vi "PH_Beckhoff_PP_PU.panel.vi"(0 "object ref":refnum<vi>, 5 "error in (no error)":errorcluster) -> (19 "error out":errorcluster)   [LabVIEW 2014, in "PH_Beckhoff_PP_PU.lvlib"]
doc: "This a GUI.\n\nLicense Agreement for this software:\n\nCopyright (C)\nGesellschaft für Schwerionenforschung, GSI\nPlanckstr. 1\n64291 Darmstadt\nGermany\n\nContact: D.Beck@gsi.de \n\nThis program is free software; you can redistribute it and/or modify it under the terms of the GNU General Public License as published by the Free Software Foundation; either version 2 of the license, or (at your option) any later version.\n\nThis program is distributed in the hope that it will be useful, but WITHOUT ANYW ARRANTY; without even the implied warranty of MERCHANTABILITY or FITNESS FOR A PARTICULAR PURPOSE. See the GNU General License for more details (http://www.gnu.org).\n\nGesellschaft für Schwerionenforschung, GSI\nPlanckstr. 1, 64291 Darmstadt, Germany\nFor all questions and ideas contact: M.Richter@gsi.de, H.Brand@gsi.de or D.Beck@gsi.de.\nLast update: 18-DEC-2002"
uses:
  PH_Beckhoff_PP_PU.lvlib
  PH_Beckhoff/PH_Beckhoff.Connectivity.ctl
  PH_Beckhoff/PH_Beckhoff.ADS Error.ctl
  PH_Beckhoff/PH_Beckhoff.Values.ctl
  PH_Beckhoff/PH_Beckhoff.Sonderklemmen Inputs.ctl
  PH_Beckhoff/PH_Beckhoff.Analog Inputs.ctl
  PH_Beckhoff/PH_Beckhoff.Scaling Type.ctl
  PH_Beckhoff/PH_Beckhoff.Analog Outputs.ctl
  PH_Beckhoff/PH_Beckhoff.Digital Inputs.ctl
  PH_Beckhoff/PH_Beckhoff.Digital Outputs.ctl
  PH_Beckhoff_PP_PU.PU Rack Type.ctl
  PH_StatusHandler/PH_StatusHandler.GUI element.ctl
  PH_PP_Common/PH_PP_Common.PSU Type.ctl
  PH_Beckhoff/PH_Beckhoff.GUI Refs.ctl
  CSCore/CSObj/CSObj.lvlib
  PH_Common/PH_Common.lvlib
  PH_Beckhoff/PH_Beckhoff.lvlib
  CSCore/CSSystem/CSSystemLib/CSSystemLib.lvlib
  PH_Class/PH_Class.lvlib
  PH_PP_Common/PH_PP_Common.lvlib
  PH_StatusHandler/PH_StatusHandler.lvlib
panel:
  in  "Tab Control":T1(tab)=enum."PUs ..."
  out "Current Values":T2
  in  "Show Info":bool
  out "configured?":bool
  out "Prdc Int [ms]":i32
  out "Connection":T9
  out "IP":string
  out "ADS Error":T10
  out "PU Rack Type":T11
  out "successfully \nreconfigured":i32=-1
  out "Trigger 2 Indicator":T13={"_Status"=0, "_triggered"=16860, "_fired"=16860, "last shot:"="no info available"} caption="_Trigger 2 ..."
  in  "_Ross close 2":bool caption="Ross 2 close"
  out "Ross 2 Indicator":T14={"_Status"=0, "_closed"=16860, "_open"=16860} caption="_Ross 2 ..."
  in  "_Device_on Ignitron 2":bool caption="Igni 2 Device-on"
  out "Ignitron 2 Indicator":T15={"_Status"=0, "_heating-on"=16860, "_water-on"=16860} caption="_Igni 2 ..."
  in  "_HV_on PSU 2":bool caption="PSU 2_HV_on"
  in  "_interlock_on PSU 2":bool caption="PSU 2_interlock_on"
  in  "_inhibit_on PSU 2":bool caption="PSU 2_inhibit_on"
  in  "_set_voltage PSU 2":dbl caption="PSU 2_voltage_set" format="%#_5g"
  out "Unit Voltage 2":string caption="V"
  out "PSU 2 Indicator":T16={"_Status"=0, "_inhibit_indicator"=16860, "_end_of_charge"=16860, "_HV_on"=16860, "_overtemperature"=16860, "_interlock_indicator"=16860, "_load_fault"=16860, "_sum_fault"=16860, "_HV_off"=16860, "_DC_ok"=16860, "_voltage_monitor"=0.0, "_current_monitor"=0.0} caption="_PSU 2 ..." {"_current_monitor" format="%#_5g"; "_voltage_monitor" format="%#_5g"}
  out "_voltage 2":dbl caption="_HV Meas 2" format="%#_7f"
  out "Unit HV Meas 2":string caption="V"
  out "Trigger 1 Indicator":T13={"_Status"=0, "_triggered"=16860, "_fired"=16860, "last shot:"="no info available"} caption="_Trigger 1 ..."
  in  "_Ross close 1":bool caption="Ross 1 close"
  out "Ross 1 Indicator":T14={"_Status"=0, "_closed"=16860, "_open"=16860} caption="_Ross 1 ..."
  in  "_Device_on Ignitron 1":bool caption="Igni 1 Device-on"
  out "Ignitron 1 Indicator":T15={"_Status"=0, "_heating-on"=16860, "_water-on"=16860} caption="_Igni 1 ..."
  in  "_HV_on PSU 1":bool caption="PSU 1_HV_on"
  in  "_interlock_on PSU 1":bool caption="PSU 1_interlock_on"
  in  "_inhibit_on PSU 1":bool caption="PSU 1_inhibit_on"
  out "PSU 1 Indicator":T16={"_Status"=0, "_inhibit_indicator"=16860, "_end_of_charge"=16860, "_HV_on"=16860, "_overtemperature"=16860, "_interlock_indicator"=16860, "_load_fault"=16860, "_sum_fault"=16860, "_HV_off"=16860, "_DC_ok"=16860, "_voltage_monitor"=0.0, "_current_monitor"=0.0} caption="_PSU 1 ..." {"_current_monitor" format="%#_5g"; "_voltage_monitor" format="%#_5g"}
  out "_voltage 1":dbl caption="_HV Meas 1" format="%#_7f"
  out "Unit HV Meas 1":string caption="V"
  in  "_set_voltage PSU 1":dbl caption="PSU 1_voltage_set" format="%#_5g"
  out "Unit Voltage 1":string caption="V"
  in  "_reset PSU 1":bool caption="PSU 1_reset"
  in  "_reset PSU 2":bool caption="PSU 2_reset"
  out "Type PSU 1":T17
  out "Type PSU 2":T17
  out "Limits 1 [V]":cluster{"Lower":dbl, "Upper":dbl}
  out "Limits 2 [V]":cluster{"Lower":dbl, "Upper":dbl}
  in  "Delete":bool
  in  "Exit":bool
  # "PCS"
  # "3.40"
  # "Pay attention! Commands are remote controlled! Handle with care!"
  # "A"
  # "V"
  # "A"
  # "V"
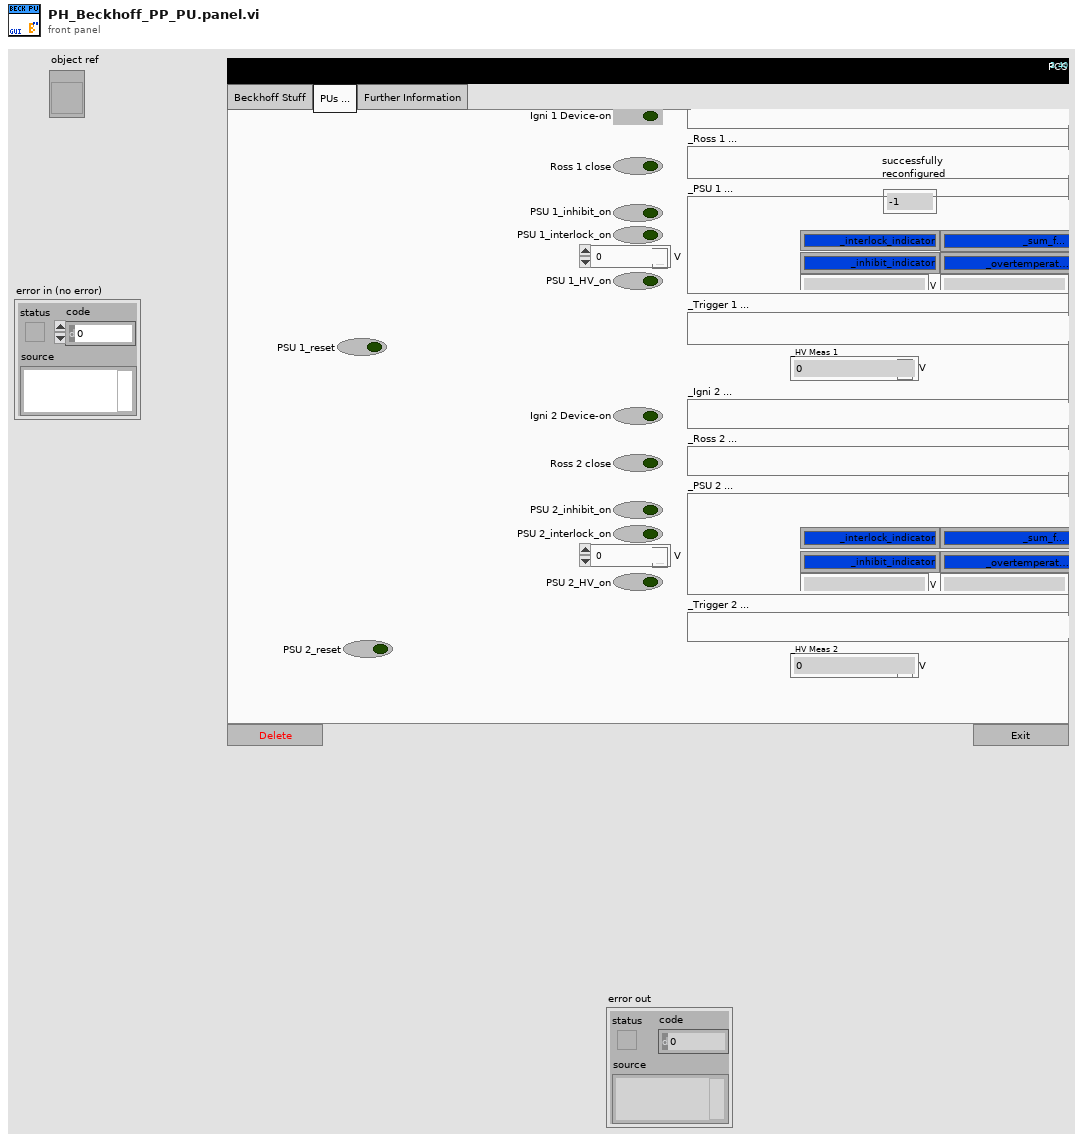
[diagram p1: front panel]
types:
  T1 = enum32{"Beckhoff Stuff", "PUs ...", "Further Information"}
  T2 = typedef "PH_Beckhoff.lvlib/PH_Beckhoff.Values.ctl" = cluster{"Sonderklemmen Inputs":T3, "Analog Inputs":T4, "Analog Outputs":T6, "Digital Inputs":T7, "Digital Outputs":T8}
  T3 = typedef "PH_Beckhoff.lvlib/PH_Beckhoff.Sonderklemmen Inputs.ctl" = cluster{"Total Length":u32, "Name":string, "Value":u64, "Quality":bool, "Service ID":i32, "Offset":u32, "Length":u32}[]
  T4 = typedef "PH_Beckhoff.lvlib/PH_Beckhoff.Analog Inputs.ctl" = cluster{"Name":string, "Value":u32, "Quality":bool, "Service ID":i32, "Sca Type":T5}[]
  T5 = typedef "PH_Beckhoff.lvlib/PH_Beckhoff.Scaling Type.ctl" = enum16{"none", "0 ... 15 Bit -> 0 ... 5", "0 ... 15 Bit -> 0 ... 10", "0 ... 15 Bit -> 0 ... 25", "0 ... 15 Bit -> 4 ... 20", "0 ... 15 Bit -> 0 ... 1", "0 ... 15 Bit -> 0 ... 20000", "0 ... 15 Bit -> 0 ... 24000"}
  T6 = typedef "PH_Beckhoff.lvlib/PH_Beckhoff.Analog Outputs.ctl" = cluster{"Name":string, "Value":u32, "Quality":bool, "Wanted Value":u32, "Service ID":i32, "Sca Type":T5}[]
  T7 = typedef "PH_Beckhoff.lvlib/PH_Beckhoff.Digital Inputs.ctl" = cluster{"Name":string, "Value":bool, "Quality":bool, "Service ID":i32, "inverted?":bool}[]
  T8 = typedef "PH_Beckhoff.lvlib/PH_Beckhoff.Digital Outputs.ctl" = cluster{"Name":string, "Value":bool, "Quality":bool, "Wanted Value":bool, "Service ID":i32, "inverted?":bool}[]
  T9 = typedef "PH_Beckhoff.lvlib/PH_Beckhoff.Connectivity.ctl" = cluster{"DLL?":bool, "Port?":bool, "Client?":bool, "Ping?":bool, "unsuccessful Pings":u32}
  T10 = typedef "PH_Beckhoff.lvlib/PH_Beckhoff.ADS Error.ctl" = cluster{"Latest Error":string, "Error List":string[]}
  T11 = typedef "PH_Beckhoff_PP_PU.lvlib/PH_Beckhoff_PP_PU.PU Rack Type.ctl" = enum16{"no Info", "PA 19mm", "PA 45mm", "MA PU 1 and 2", "MA PU 3 and 4", "MA PU 5 and 6", "MA FR and PILC"}
  T12 = typedef "PH_StatusHandler.lvlib/PH_StatusHandler.GUI element.ctl" = u16
  T13 = cluster{"_Status":T12, "_triggered":u32, "_fired":u32, "last shot:":string}
  T14 = cluster{"_Status":T12, "_closed":u32, "_open":u32}
  T15 = cluster{"_Status":T12, "_heating-on":u32, "_water-on":u32}
  T16 = cluster{"_Status":T12, "_inhibit_indicator":u32, "_end_of_charge":u32, "_HV_on":u32, "_overtemperature":u32, "_interlock_indicator":u32, "_load_fault":u32, "_sum_fault":u32, "_HV_off":u32, "_DC_ok":u32, "_voltage_monitor":dbl, "_current_monitor":dbl}
  T17 = typedef "PH_PP_Common.lvlib/PH_PP_Common.PSU Type.ctl" = enum16{"none", "Maxwell Standard", "DEL", "Maxwell ALE", "Continuum 601k"}
  T18 = typedef "PH_Beckhoff.lvlib/PH_Beckhoff.GUI Refs.ctl" = cluster{"ADS Error":refnum<vi>, "Values":refnum<vi>, "configured?":refnum<vi>, "Connection":refnum<vi>, "IP":refnum<vi>, "Prdc Int [ms]":refnum<vi>}
  T19 = typedef "PH_Beckhoff.lvlib/PH_Beckhoff.i attribute.ctl" = cluster{"GUI Refs":T18, "operation?":bool, "Default Prdc Interval":i32, "Connection":T9, "AMS Net ID":T20, "Klemmencluster: # of":T21, "Values":T2, "IP":string, "Description":string, "configured?":bool, "Change Manager":cluster{"Detemination wanted?":bool, "Values changed at":cluster{"Sonderklemmen Inputs":i32[], "Analog Inputs":i32[], "Analog Outputs":i32[], "Digital Inputs":i32[], "Digital Outputs":i32[]}}, "Difference to handle an analog input as change":u32}
  T20 = typedef "Beckhoff - Driver np.lvlib/Beckhoff Access.ctl" = cluster{"DLL path":path, "AMS Net ID":cluster{"1st # of IP":u8, "2nd # of IP":u8, "3rd # of IP":u8, "4th # of IP":u8, "In Port":u8, "Out Port":u8}}
  T21 = typedef "Beckhoff - Driver np.lvlib/Klemmendeclarer.ctl" = cluster{"Offset due to Sonderklemms":u32, "analog Inputs":u32, "analog Outputs":u32, "digital Input Bits":u32, "digital Output Bits":u32}
  T22 = typedef "PH_PP_Common.lvlib/PH_PP_Common.PUs.ctl" = enum16{"no Info", "PA-19mm-1", "PA-19mm-2", "PA-45mm-PILC", "PA-45mm-MAIN", "MA-PU-1", "MA-PU-2", "MA-PU-3", "MA-PU-4", "MA-PU-5", "MA-PU-6", "MA-FR", "MA-PILC", "PA-45mm-DP"}
  T23 = typedef "PH_Beckhoff_PP_PU.lvlib/PH_Beckhoff_PP_PU.i attribute.ctl" = cluster{"HV Meas":cluster{"Input GUI Ref":refnum<vi>, "Voltage Service ID":i32, "Voltage [V]":dbl, "Quality":bool, "# in Data":i32}[], "Trigger":cluster{"Status":cluster{"GUI Ref":refnum<vi>, "Status Service ID":i32, "Status":T24}, "last shot:":cluster{"GUI Ref":refnum<vi>, "Service ID":i32, "Time":string}, "DIs":cluster{"triggered":cluster{"GUI Ref":refnum<vi>, "# in Data":i32}, "fired":cluster{"GUI Ref":refnum<vi>, "# in Data":i32}}, "GUI Ref Indicator":refnum<vi>}[], "RR":cluster{"Status":cluster{"GUI Ref":refnum<vi>, "Status Service ID":i32, "Status":T24}, "DIs":cluster{"closed":cluster{"GUI Ref":refnum<vi>, "# in Data":i32}, "open":cluster{"GUI Ref":refnum<vi>, "# in Data":i32}}, "Close":cluster{"GUI Ref":refnum<vi>, "# in Data":i32}, "GUI Ref Indicator":refnum<vi>}[], "Igni":cluster{"Status":cluster{"GUI Ref":refnum<vi>, "Status Service ID":i32, "Status":T24}, "DIs":cluster{"heating on":cluster{"GUI Ref":refnum<vi>, "# in Data":i32}, "water on":cluster{"GUI Ref":refnum<vi>, "# in Data":i32}}, "Device on":cluster{"GUI Ref":refnum<vi>, "# in Data":i32}, "GUI Ref Indicator":refnum<vi>}[], "PSU":cluster{"Status":cluster{"GUI Ref":refnum<vi>, "Status Service ID":i32, "Status":T24}, "Limit Service ID":i32, "DIs":cluster{"inhibit":cluster{"GUI Ref":refnum<vi>, "# in Data":i32}, "end of charge":cluster{"GUI Ref":refnum<vi>, "# in Data":i32}, "HV on":cluster{"GUI Ref":refnum<vi>, "# in Data":i32}, "overtemp":cluster{"GUI Ref":refnum<vi>, "# in Data":i32}, "interlock":cluster{"GUI Ref":refnum<vi>, "# in Data":i32}, "load fault":cluster{"GUI Ref":refnum<vi>, "# in Data":i32}, "sum fault":cluster{"GUI Ref":refnum<vi>, "# in Data":i32}, "HV off":cluster{"GUI Ref":refnum<vi>, "# in Data":i32}, "DC ok":cluster{"GUI Ref":refnum<vi>, "# in Data":i32}}, "AIs":cluster{"voltage":cluster{"GUI Ref":refnum<vi>, "# in Data":i32}, "current":cluster{"GUI Ref":refnum<vi>, "# in Data":i32}}, "DAs":cluster{"inhibit":cluster{"GUI Ref":refnum<vi>, "# in Data":i32}, "interlock":cluster{"GUI Ref":refnum<vi>, "# in Data":i32}, "HV on":cluster{"GUI Ref":refnum<vi>, "# in Data":i32}, "Reset":cluster{"GUI Ref":refnum<vi>, "# in Data":i32}}, "AAs":cluster{"Voltage to set":cluster{"GUI Ref":refnum<vi>, "# in Data":i32}}, "GUI Ref Indicator":refnum<vi>}[], "reconfigured":cluster{"?":bool, "GUI Ref":refnum<vi>}, "PU Rack Type":T11, "HV Meas Info":T25, "PSU Info":T26}
  T24 = typedef "PH_StatusHandler.lvlib/PH_StatusHandler.Status.ctl" = i16
  T25 = typedef "PH_Beckhoff_PP_PU.lvlib/PH_Beckhoff_PP_PU.HV Meas Info.ctl" = cluster{"Period Time [s]":dbl, "Subtractor 1 [Hz]":dbl, "Devider 1 [Hz/kV]":dbl, "Subtractor 2 [Hz]":dbl, "Devider 2 [Hz/kV]":dbl}
  T26 = typedef "PH_Beckhoff_PP_PU.lvlib/PH_Beckhoff_PP_PU.PSU Info.ctl" = cluster{"Limits 1 [V]":cluster{"Lower":dbl, "Upper":dbl}, "Limits 2 [V]":cluster{"Lower":dbl, "Upper":dbl}}
  T27 = cluster{"Status":cluster{"GUI Ref":refnum<vi>, "Status Service ID":i32, "Status":T24}, "DIs":cluster{"heating on":cluster{"GUI Ref":refnum<vi>, "# in Data":i32}, "water on":cluster{"GUI Ref":refnum<vi>, "# in Data":i32}}, "Device on":cluster{"GUI Ref":refnum<vi>, "# in Data":i32}, "GUI Ref Indicator":refnum<vi>}[]
  T28 = cluster{"Status":cluster{"GUI Ref":refnum<vi>, "Status Service ID":i32, "Status":T24}, "DIs":cluster{"closed":cluster{"GUI Ref":refnum<vi>, "# in Data":i32}, "open":cluster{"GUI Ref":refnum<vi>, "# in Data":i32}}, "Close":cluster{"GUI Ref":refnum<vi>, "# in Data":i32}, "GUI Ref Indicator":refnum<vi>}[]
  T29 = cluster{"Status":cluster{"GUI Ref":refnum<vi>, "Status Service ID":i32, "Status":T24}, "last shot:":cluster{"GUI Ref":refnum<vi>, "Service ID":i32, "Time":string}, "DIs":cluster{"triggered":cluster{"GUI Ref":refnum<vi>, "# in Data":i32}, "fired":cluster{"GUI Ref":refnum<vi>, "# in Data":i32}}, "GUI Ref Indicator":refnum<vi>}[]
  T30 = cluster{"Input GUI Ref":refnum<vi>, "Voltage Service ID":i32, "Voltage [V]":dbl, "Quality":bool, "# in Data":i32}[]
  T31 = cluster{"Status":cluster{"GUI Ref":refnum<vi>, "Status Service ID":i32, "Status":T24}, "Limit Service ID":i32, "DIs":cluster{"inhibit":cluster{"GUI Ref":refnum<vi>, "# in Data":i32}, "end of charge":cluster{"GUI Ref":refnum<vi>, "# in Data":i32}, "HV on":cluster{"GUI Ref":refnum<vi>, "# in Data":i32}, "overtemp":cluster{"GUI Ref":refnum<vi>, "# in Data":i32}, "interlock":cluster{"GUI Ref":refnum<vi>, "# in Data":i32}, "load fault":cluster{"GUI Ref":refnum<vi>, "# in Data":i32}, "sum fault":cluster{"GUI Ref":refnum<vi>, "# in Data":i32}, "HV off":cluster{"GUI Ref":refnum<vi>, "# in Data":i32}, "DC ok":cluster{"GUI Ref":refnum<vi>, "# in Data":i32}}, "AIs":cluster{"voltage":cluster{"GUI Ref":refnum<vi>, "# in Data":i32}, "current":cluster{"GUI Ref":refnum<vi>, "# in Data":i32}}, "DAs":cluster{"inhibit":cluster{"GUI Ref":refnum<vi>, "# in Data":i32}, "interlock":cluster{"GUI Ref":refnum<vi>, "# in Data":i32}, "HV on":cluster{"GUI Ref":refnum<vi>, "# in Data":i32}, "Reset":cluster{"GUI Ref":refnum<vi>, "# in Data":i32}}, "AAs":cluster{"Voltage to set":cluster{"GUI Ref":refnum<vi>, "# in Data":i32}}, "GUI Ref Indicator":refnum<vi>}[]
  T32 = cluster{"Status":cluster{"GUI Ref":refnum<vi>, "Status Service ID":i32, "Status":T24}, "Limit Service ID":i32, "DIs":cluster{"inhibit":cluster{"GUI Ref":refnum<vi>, "# in Data":i32}, "end of charge":cluster{"GUI Ref":refnum<vi>, "# in Data":i32}, "HV on":cluster{"GUI Ref":refnum<vi>, "# in Data":i32}, "overtemp":cluster{"GUI Ref":refnum<vi>, "# in Data":i32}, "interlock":cluster{"GUI Ref":refnum<vi>, "# in Data":i32}, "load fault":cluster{"GUI Ref":refnum<vi>, "# in Data":i32}, "sum fault":cluster{"GUI Ref":refnum<vi>, "# in Data":i32}, "HV off":cluster{"GUI Ref":refnum<vi>, "# in Data":i32}, "DC ok":cluster{"GUI Ref":refnum<vi>, "# in Data":i32}}, "AIs":cluster{"voltage":cluster{"GUI Ref":refnum<vi>, "# in Data":i32}, "current":cluster{"GUI Ref":refnum<vi>, "# in Data":i32}}, "DAs":cluster{"inhibit":cluster{"GUI Ref":refnum<vi>, "# in Data":i32}, "interlock":cluster{"GUI Ref":refnum<vi>, "# in Data":i32}, "HV on":cluster{"GUI Ref":refnum<vi>, "# in Data":i32}, "Reset":cluster{"GUI Ref":refnum<vi>, "# in Data":i32}}, "AAs":cluster{"Voltage to set":cluster{"GUI Ref":refnum<vi>, "# in Data":i32}}, "GUI Ref Indicator":refnum<vi>}
  T33 = cluster{"Status":cluster{"GUI Ref":refnum<vi>, "Status Service ID":i32, "Status":T24}, "DIs":cluster{"heating on":cluster{"GUI Ref":refnum<vi>, "# in Data":i32}, "water on":cluster{"GUI Ref":refnum<vi>, "# in Data":i32}}, "Device on":cluster{"GUI Ref":refnum<vi>, "# in Data":i32}, "GUI Ref Indicator":refnum<vi>}
  T34 = cluster{"Status":cluster{"GUI Ref":refnum<vi>, "Status Service ID":i32, "Status":T24}, "DIs":cluster{"closed":cluster{"GUI Ref":refnum<vi>, "# in Data":i32}, "open":cluster{"GUI Ref":refnum<vi>, "# in Data":i32}}, "Close":cluster{"GUI Ref":refnum<vi>, "# in Data":i32}, "GUI Ref Indicator":refnum<vi>}
  T35 = cluster{"Status":cluster{"GUI Ref":refnum<vi>, "Status Service ID":i32, "Status":T24}, "last shot:":cluster{"GUI Ref":refnum<vi>, "Service ID":i32, "Time":string}, "DIs":cluster{"triggered":cluster{"GUI Ref":refnum<vi>, "# in Data":i32}, "fired":cluster{"GUI Ref":refnum<vi>, "# in Data":i32}}, "GUI Ref Indicator":refnum<vi>}
  T36 = cluster{"Input GUI Ref":refnum<vi>, "Voltage Service ID":i32, "Voltage [V]":dbl, "Quality":bool, "# in Data":i32}
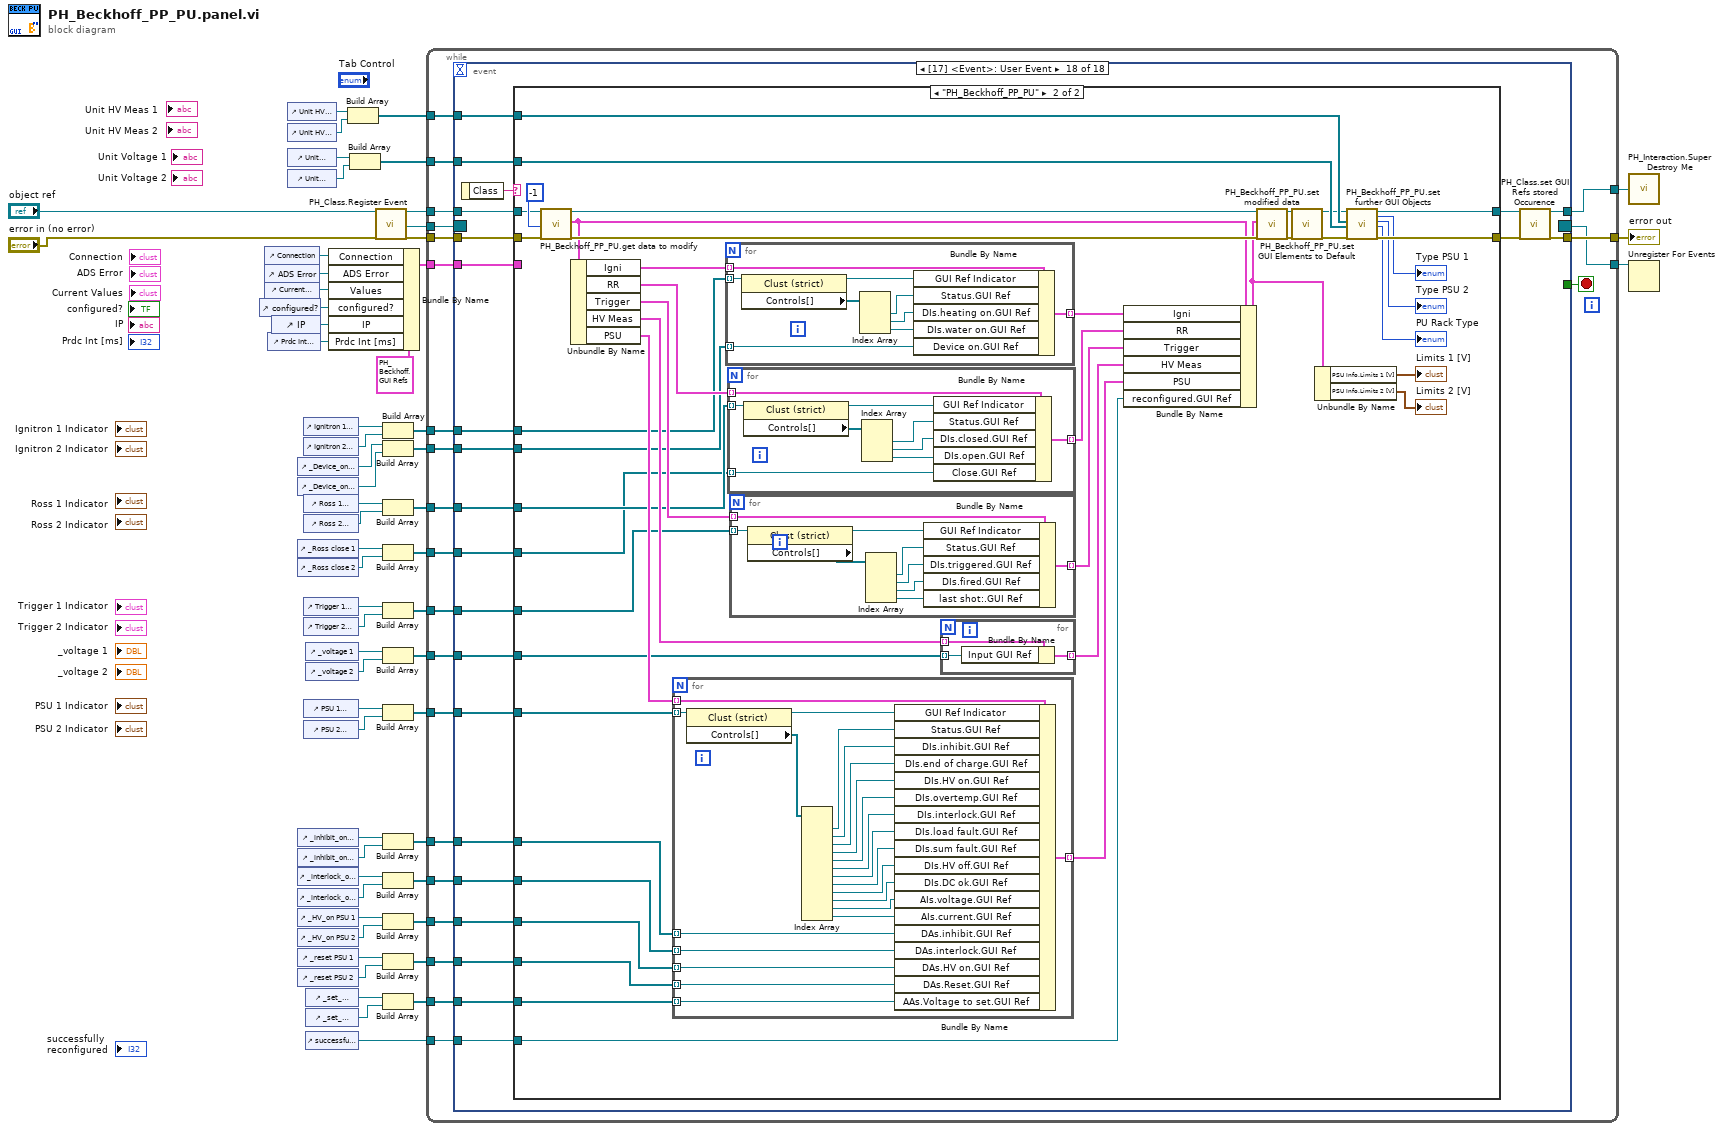
[diagram p0: block diagram]
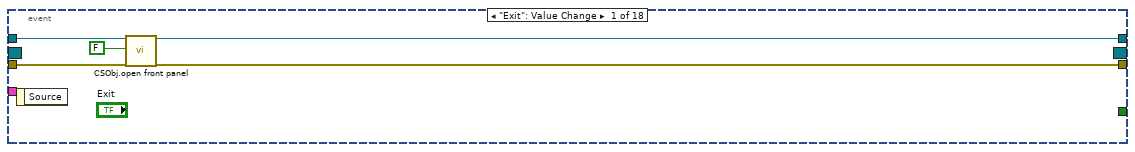
[diagram p2: hidden frame]
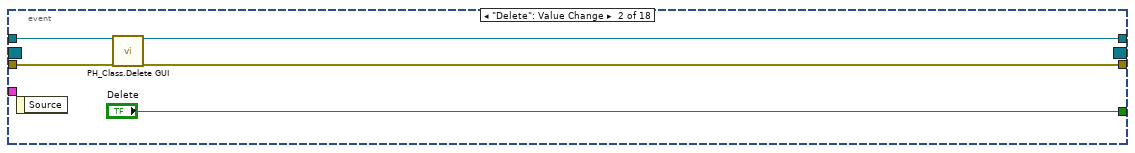
[diagram p3: hidden frame]
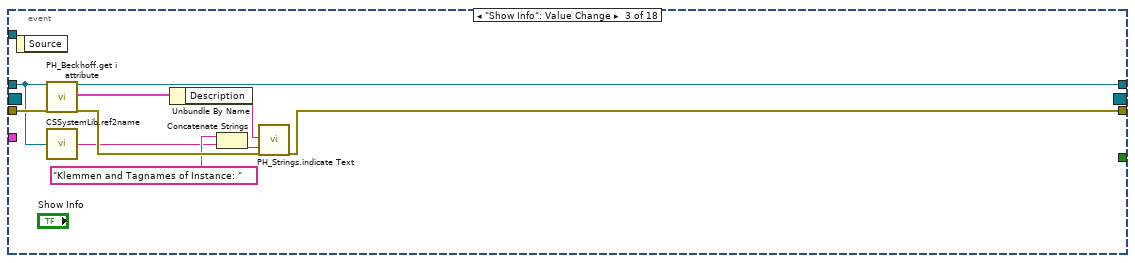
[diagram p4: hidden frame]
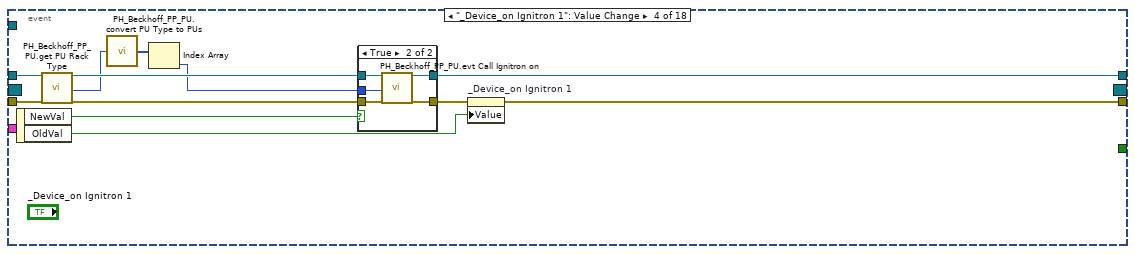
[diagram p5: hidden frame]
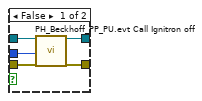
[diagram p6: hidden frame]
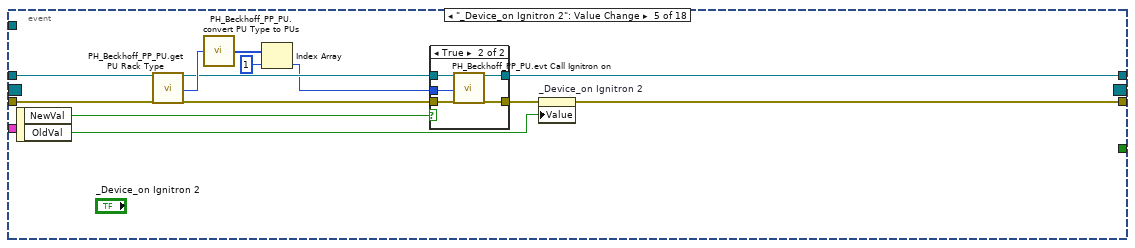
[diagram p7: hidden frame]
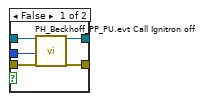
[diagram p8: hidden frame]
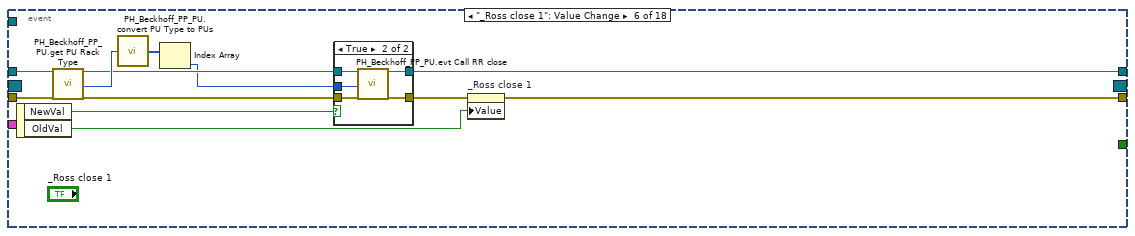
[diagram p9: hidden frame]
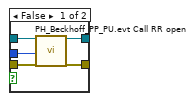
[diagram p10: hidden frame]
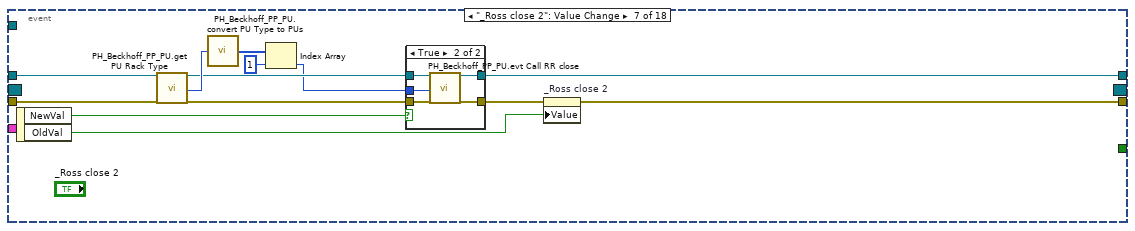
[diagram p11: hidden frame]
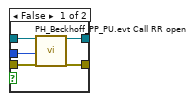
[diagram p12: hidden frame]
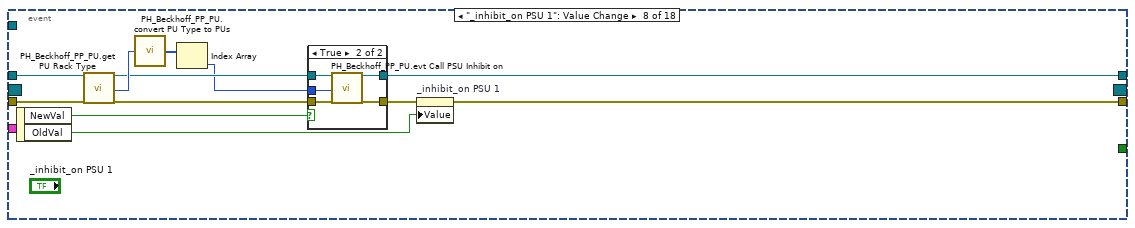
[diagram p13: hidden frame]
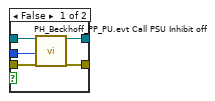
[diagram p14: hidden frame]
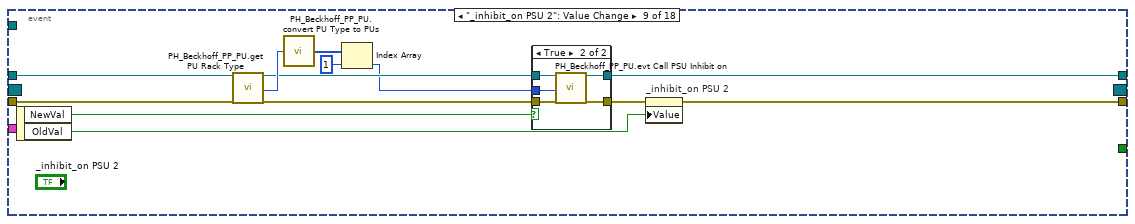
[diagram p15: hidden frame]
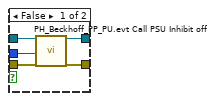
[diagram p16: hidden frame]
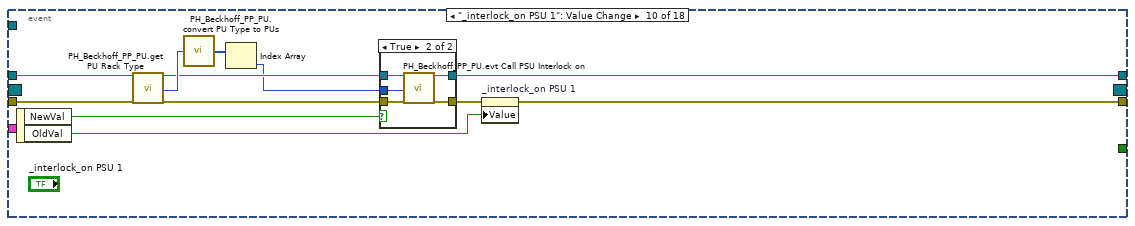
[diagram p17: hidden frame]
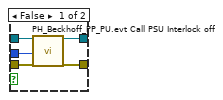
[diagram p18: hidden frame]
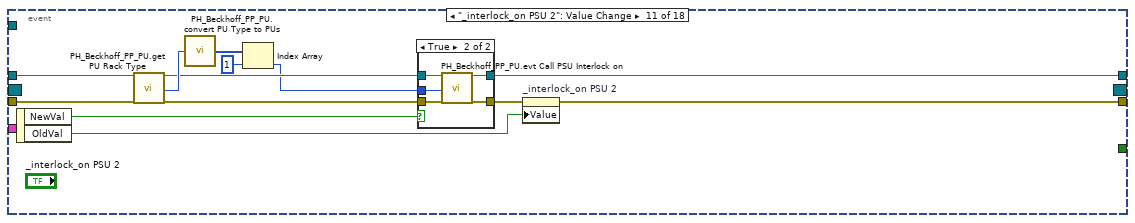
[diagram p19: hidden frame]
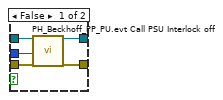
[diagram p20: hidden frame]
diagram:
  n1 = control-ref of="configured?"() -> (w46:refnum<vi>)
  n2 = control-ref of="Connection"() -> (w57:refnum<vi>)
  n3 = control-ref of="ADS Error"() -> (w56:refnum<vi>)
  n4 = control-ref of="Current Values"() -> (w55:refnum<vi>)
  n5 = control-ref of="Prdc Int [ms]"() -> (w5:refnum<vi>)
  n6 = control-ref of="IP"() -> (w6:refnum<vi>)
  n7 = control-ref of="Unit HV Meas 1"() -> (w39:refnum<vi>)
  n8 = control-ref of="Unit HV Meas 2"() -> (w38:refnum<vi>)
  n9 = control-ref of="Unit Voltage 1"() -> (w37:refnum<vi>)
  n10 = control-ref of="Unit Voltage 2"() -> (w36:refnum<vi>)
  n11 = control-ref of="_Device_on Ignitron 1"() -> (w48:refnum<vi>)
  n12 = control-ref of="_Device_on Ignitron 2"() -> (w47:refnum<vi>)
  n13 = control-ref of="_Ross close 1"() -> (w43:refnum<vi>)
  n14 = control-ref of="_Ross close 2"() -> (w42:refnum<vi>)
  n15 = control-ref of="_inhibit_on PSU 1"() -> (w35:refnum<vi>)
  n16 = control-ref of="_inhibit_on PSU 2"() -> (w34:refnum<vi>)
  n17 = control-ref of="_interlock_on PSU 1"() -> (w33:refnum<vi>)
  n18 = control-ref of="_interlock_on PSU 2"() -> (w32:refnum<vi>)
  n19 = control-ref of="_HV_on PSU 1"() -> (w31:refnum<vi>)
  n20 = control-ref of="_HV_on PSU 2"() -> (w30:refnum<vi>)
  n21 = control-ref of="_reset PSU 1"() -> (w29:refnum<vi>)
  n22 = control-ref of="_reset PSU 2"() -> (w28:refnum<vi>)
  n23 = control-ref of="Ignitron 1 Indicator"() -> (w50:refnum<vi>)
  n24 = control-ref of="Ignitron 2 Indicator"() -> (w49:refnum<vi>)
  n25 = control-ref of="Ross 1 Indicator"() -> (w45:refnum<vi>)
  n26 = control-ref of="Ross 2 Indicator"() -> (w44:refnum<vi>)
  n27 = control-ref of="Trigger 1 Indicator"() -> (w41:refnum<vi>)
  n28 = control-ref of="Trigger 2 Indicator"() -> (w40:refnum<vi>)
  n29 = control-ref of="PSU 1 Indicator"() -> (w52:refnum<vi>)
  n30 = control-ref of="PSU 2 Indicator"() -> (w51:refnum<vi>)
  n31 = control-ref of="_voltage 1"() -> (w54:refnum<vi>)
  n32 = control-ref of="_voltage 2"() -> (w53:refnum<vi>)
  n33 = control-ref of="_set_voltage PSU 1"() -> (w27:refnum<vi>)
  n34 = control-ref of="_set_voltage PSU 2"() -> (w26:refnum<vi>)
  n35 = control-ref of="successfully \nreconfigured"() -> (w8:refnum<vi>)
  n36 = Bundle By Name(cluster=T18 {"ADS Error"=refnum, "Values"=refnum, "configured?"=refnum, "Connection"=refnum, "IP"=refnum, "Prdc Int [ms]"=refnum} ("GUI Dummy"), "Connection"=w57, "ADS Error"=w56, "Values"=w55, "configured?"=w46, "IP"=w6, "Prdc Int [ms]"=w5) -> (w7:T18)
  n37 = Build Array(w39, w38) -> (w1:refnum<vi>[])
  n38 = Build Array(w37, w36) -> (w2:refnum<vi>[])
  n39 = call "PH_Class.Register Event.vi"("i ref in"="object ref", "error in (no error)"="error in (no error)") -> ("i ref out"=w24:refnum<vi>, "Event Registration Refnum"=w22:refnum<event-registration>, "error out"=w23:errorcluster)  [unwired: 15 in]
  n40 = Build Array(w50, w49) -> (w20:refnum<vi>[])
  n41 = Build Array(w48, w47) -> (w19:refnum<vi>[])
  n42 = Build Array(w45, w44) -> (w18:refnum<vi>[])
  n43 = Build Array(w43, w42) -> (w17:refnum<vi>[])
  n44 = Build Array(w41, w40) -> (w16:refnum<vi>[])
  n45 = Build Array(w54, w53) -> (w15:refnum<vi>[])
  n46 = Build Array(w52, w51) -> (w14:refnum<vi>[])
  n47 = Build Array(w35, w34) -> (w13:refnum<vi>[])
  n48 = Build Array(w33, w32) -> (w12:refnum<vi>[])
  n49 = Build Array(w31, w30) -> (w11:refnum<vi>[])
  n50 = Build Array(w29, w28) -> (w10:refnum<vi>[])
  n51 = Build Array(w27, w26) -> (w9:refnum<vi>[])
  n52 = while {
    tunnel: w24 -> [w79]
    tunnel: [w78] -> w59
    tunnel: w23 -> [w81]
    tunnel: [w80] -> w58
    tunnel: w22 -> [w77]
    tunnel: [w76] -> w21
    tunnel: w20 -> [w75]
    tunnel: w19 -> [w74]
    tunnel: w18 -> [w73]
    tunnel: w17 -> [w72]
    tunnel: w16 -> [w71]
    tunnel: w15 -> [w70]
    tunnel: w14 -> [w69]
    tunnel: w13 -> [w68]
    tunnel: w12 -> [w67]
    tunnel: w11 -> [w66]
    tunnel: w10 -> [w65]
    tunnel: w9 -> [w64]
    tunnel: w8 -> [w63]
    tunnel: w7 -> [w62]
    tunnel: w2 -> [w61]
    tunnel: w1 -> [w60]
    stop <- w82 stop-if-true
    n53 = event shown="[17] <Event>: User Event" {
      selector: w77 -> [_ _ _ _ _ _ _ _ _ _ _ _ _ _ _ _ _ _]
      dyn-events: [_ _ _ _ _ _ _ _ _ _ _ _ _ _ _ _ _ _] -> w76
      timeout: _ -> [_ _ _ _ _ _ _ _ _ _ _ _ _ _ _ _ _ _]
      tunnel: [_ "Delete" _ _ _ _ _ _ _ _ _ _ _ _ _ _ _ _] -> w82
      tunnel: w79 -> [w84 w89 w93 w107 w129 w149 w174 w195 w219 w242 w264 w287 w309 w332 w354 w376 w394 w428]
      tunnel: w81 -> [w87 w91 w102 w111 w128 w148 w173 w197 w218 w241 w263 w286 w308 w331 w353 w378 w395 w427]
      tunnel: [w86 w90 w99 w114 w133 w155 w179 w202 w226 w248 w271 w294 w316 w336 w359 w385 w405 w410] -> w80
      tunnel: [w83 w88 w101 w109 w136 w158 w181 w204 w224 w246 w268 w292 w313 w338 w361 w388 w402 w408] -> w78
      tunnel: w75 -> [_ _ _ _ _ _ _ _ _ _ _ _ _ _ _ _ _ w424]
      tunnel: w74 -> [_ _ _ _ _ _ _ _ _ _ _ _ _ _ _ _ _ w423]
      tunnel: w73 -> [_ _ _ _ _ _ _ _ _ _ _ _ _ _ _ _ _ w422]
      tunnel: w72 -> [_ _ _ _ _ _ _ _ _ _ _ _ _ _ _ _ _ w421]
      tunnel: w71 -> [_ _ _ _ _ _ _ _ _ _ _ _ _ _ _ _ _ w420]
      tunnel: w70 -> [_ _ _ _ _ _ _ _ _ _ _ _ _ _ _ _ _ w419]
      tunnel: w69 -> [_ _ _ _ _ _ _ _ _ _ _ _ _ _ _ _ _ w418]
      tunnel: w68 -> [_ _ _ _ _ _ _ _ _ _ _ _ _ _ _ _ _ w417]
      tunnel: w67 -> [_ _ _ _ _ _ _ _ _ _ _ _ _ _ _ _ _ w416]
      tunnel: w66 -> [_ _ _ _ _ _ _ _ _ _ _ _ _ _ _ _ _ w415]
      tunnel: w65 -> [_ _ _ _ _ _ _ _ _ _ _ _ _ _ _ _ _ w414]
      tunnel: w64 -> [_ _ _ _ _ _ _ _ _ _ _ _ _ _ _ _ _ w413]
      tunnel: w63 -> [_ _ _ _ _ _ _ _ _ _ _ _ _ _ _ _ _ w412]
      tunnel: w62 -> [_ _ _ _ _ _ _ _ _ _ _ _ _ _ _ _ _ w411]
      tunnel: w61 -> [_ _ _ _ _ _ _ _ _ _ _ _ _ _ _ _ _ w407]
      tunnel: w60 -> [_ _ _ _ _ _ _ _ _ _ _ _ _ _ _ _ _ w406]
      event "Exit": Value Change {
        n54 = event-data() -> ()  [unwired: 1 in, 1 out]
        n55 = call "CSObj.open front panel.vi"("i ref in"=w84, "frontPanelOpen"=FALSE ("front panel open"), "error in (no error)"=w87) -> ("i ref out"=w83:refnum<vi>, "error out"=w86:errorcluster)  [unwired: 15 in]
      }
      event "Delete": Value Change {
        n56 = event-data() -> ()  [unwired: 1 in, 1 out]
        n57 = call "PH_Class.Delete GUI.vi"("VI in"=w89, "error in (no error)"=w91) -> ("VI out"=w88:refnum<vi>, "error out"=w90:errorcluster)  [unwired: 16 in]
      }
      event "Show Info": Value Change {
        n58 = event-data() -> ()  [unwired: 1 in, 1 out]
        n59 = call "PH_Beckhoff.get i attribute.vi"("i ref in"=w93, "error in (no error)"=w102) -> ("i ref out"=w101:refnum<vi>, "i attribute"=w98:T19, "error out"=w100:errorcluster)  [unwired: 15 in]
        n60 = call "CSSystemLib.ref2name.vi"("obj refnum"=w93) -> ("name"=w94:string)
        n61 = Unbundle By Name(w98) -> ("Description"=w97:string)
        n62 = Concatenate Strings("Klemmen and Tagnames of Instance: " ("Caption.Text"), w94) -> (w95:string)
        n63 = call "PH_Strings.indicate Text.vi"("String to show"=w97, "Caption.Text"=w95, "error in (no error)"=w100) -> ("error out"=w99:errorcluster)  [unwired: 16 in]
      }
      event "_Device_on Ignitron 1": Value Change {
        n64 = event-data() -> ("NewVal"=w112:bool, "OldVal"=w113:bool)  [unwired: 1 in]
        n65 = call "PH_Beckhoff_PP_PU.get PU Rack Type.vi"("VI in"=w107, "error in (no error)"=w111) -> ("VI out"=w106:refnum<vi>, "PU Rack Type"=w105:T11, "error out"=w108:errorcluster)  [unwired: 15 in]
        n66 = call "PH_Beckhoff_PP_PU.convert PU Type to PUs.vi"("PU Type"=w105) -> ("PUs"=w104:T22[])
        n67 = Index Array(array=w104) -> (element=w103:T22)  [unwired: 1 in]
        n68 = case shown="True" w112 {
          tunnel: w106 -> [w119 w124]
          tunnel: [w118 w123] -> w109
          tunnel: w108 -> [w117 w122]
          tunnel: [w116 w121] -> w110
          tunnel: w103 -> [w115 w120]
          frame False {
            n69 = call "PH_Beckhoff_PP_PU.evt Call Ignitron off.vi"("i ref in"=w119, "PU"=w115, "error in"=w117) -> ("i ref out"=w118:refnum<vi>, "error out"=w116:errorcluster)  [unwired: 15 in]
          }
          frame True {
            n70 = call "PH_Beckhoff_PP_PU.evt Call Ignitron on.vi"("i ref in"=w124, "PU"=w120, "error in"=w122) -> ("i ref out"=w123:refnum<vi>, "error out"=w121:errorcluster)  [unwired: 15 in]
          }
        }
        n71 = property on="_Device_on Ignitron 1" class="Bool (strict)"(error in=w110, "Value"=w113) -> (error out=w114:errorcluster)  [unwired: 1 in, 1 out]
      }
      event "_Device_on Ignitron 2": Value Change {
        n72 = event-data() -> ("NewVal"=w137:bool, "OldVal"=w134:bool)  [unwired: 1 in]
        n73 = call "PH_Beckhoff_PP_PU.get PU Rack Type.vi"("VI in"=w129, "error in (no error)"=w128) -> ("VI out"=w126:refnum<vi>, "PU Rack Type"=w132:T11, "error out"=w127:errorcluster)  [unwired: 15 in]
        n74 = call "PH_Beckhoff_PP_PU.convert PU Type to PUs.vi"("PU Type"=w132) -> ("PUs"=w131:T22[])
        n75 = Index Array(array=w131, index=1) -> (element=w125:T22)
        n76 = case shown="True" w137 {
          tunnel: w126 -> [w142 w147]
          tunnel: [w141 w146] -> w136
          tunnel: w127 -> [w140 w145]
          tunnel: [w139 w144] -> w135
          tunnel: w125 -> [w138 w143]
          frame False {
            n77 = call "PH_Beckhoff_PP_PU.evt Call Ignitron off.vi"("i ref in"=w142, "PU"=w138, "error in"=w140) -> ("i ref out"=w141:refnum<vi>, "error out"=w139:errorcluster)  [unwired: 15 in]
          }
          frame True {
            n78 = call "PH_Beckhoff_PP_PU.evt Call Ignitron on.vi"("i ref in"=w147, "PU"=w143, "error in"=w145) -> ("i ref out"=w146:refnum<vi>, "error out"=w144:errorcluster)  [unwired: 15 in]
          }
        }
        n79 = property on="_Device_on Ignitron 2" class="Bool (strict)"(error in=w135, "Value"=w134) -> (error out=w133:errorcluster)  [unwired: 1 in, 1 out]
      }
      event "_Ross close 1": Value Change {
        n80 = event-data() -> ("NewVal"=w159:bool, "OldVal"=w157:bool)  [unwired: 1 in]
        n81 = call "PH_Beckhoff_PP_PU.get PU Rack Type.vi"("VI in"=w149, "error in (no error)"=w148) -> ("VI out"=w152:refnum<vi>, "PU Rack Type"=w154:T11, "error out"=w150:errorcluster)  [unwired: 15 in]
        n82 = call "PH_Beckhoff_PP_PU.convert PU Type to PUs.vi"("PU Type"=w154) -> ("PUs"=w153:T22[])
        n83 = Index Array(array=w153) -> (element=w151:T22)  [unwired: 1 in]
        n84 = case shown="True" w159 {
          tunnel: w152 -> [w164 w169]
          tunnel: [w163 w168] -> w158
          tunnel: w150 -> [w162 w167]
          tunnel: [w161 w166] -> w156
          tunnel: w151 -> [w160 w165]
          frame False {
            n85 = call "PH_Beckhoff_PP_PU.evt Call RR open.vi"("i ref in"=w164, "PU"=w160, "error in"=w162) -> ("i ref out"=w163:refnum<vi>, "error out"=w161:errorcluster)  [unwired: 15 in]
          }
          frame True {
            n86 = call "PH_Beckhoff_PP_PU.evt Call RR close.vi"("i ref in"=w169, "PU"=w165, "error in"=w167) -> ("i ref out"=w168:refnum<vi>, "error out"=w166:errorcluster)  [unwired: 15 in]
          }
        }
        n87 = property on="_Ross close 1" class="Bool (strict)"(error in=w156, "Value"=w157) -> (error out=w155:errorcluster)  [unwired: 1 in, 1 out]
      }
      event "_Ross close 2": Value Change {
        n88 = event-data() -> ("NewVal"=w182:bool, "OldVal"=w178:bool)  [unwired: 1 in]
        n89 = call "PH_Beckhoff_PP_PU.get PU Rack Type.vi"("VI in"=w174, "error in (no error)"=w173) -> ("VI out"=w171:refnum<vi>, "PU Rack Type"=w177:T11, "error out"=w172:errorcluster)  [unwired: 15 in]
        n90 = call "PH_Beckhoff_PP_PU.convert PU Type to PUs.vi"("PU Type"=w177) -> ("PUs"=w176:T22[])
        n91 = Index Array(array=w176, index=1) -> (element=w170:T22)
        n92 = case shown="True" w182 {
          tunnel: w171 -> [w187 w192]
          tunnel: [w186 w191] -> w181
          tunnel: w172 -> [w185 w190]
          tunnel: [w184 w189] -> w180
          tunnel: w170 -> [w183 w188]
          frame False {
            n93 = call "PH_Beckhoff_PP_PU.evt Call RR open.vi"("i ref in"=w187, "PU"=w183, "error in"=w185) -> ("i ref out"=w186:refnum<vi>, "error out"=w184:errorcluster)  [unwired: 15 in]
          }
          frame True {
            n94 = call "PH_Beckhoff_PP_PU.evt Call RR close.vi"("i ref in"=w192, "PU"=w188, "error in"=w190) -> ("i ref out"=w191:refnum<vi>, "error out"=w189:errorcluster)  [unwired: 15 in]
          }
        }
        n95 = property on="_Ross close 2" class="Bool (strict)"(error in=w180, "Value"=w178) -> (error out=w179:errorcluster)  [unwired: 1 in, 1 out]
      }
      event "_inhibit_on PSU 1": Value Change {
        n96 = event-data() -> ("NewVal"=w200:bool, "OldVal"=w201:bool)  [unwired: 1 in]
        n97 = call "PH_Beckhoff_PP_PU.get PU Rack Type.vi"("VI in"=w195, "error in (no error)"=w197) -> ("VI out"=w194:refnum<vi>, "PU Rack Type"=w199:T11, "error out"=w196:errorcluster)  [unwired: 15 in]
        n98 = call "PH_Beckhoff_PP_PU.convert PU Type to PUs.vi"("PU Type"=w199) -> ("PUs"=w198:T22[])
        n99 = Index Array(array=w198) -> (element=w193:T22)  [unwired: 1 in]
        n100 = case shown="True" w200 {
          tunnel: w194 -> [w209 w214]
          tunnel: [w208 w213] -> w204
          tunnel: w196 -> [w207 w212]
          tunnel: [w206 w211] -> w203
          tunnel: w193 -> [w205 w210]
          frame False {
            n101 = call "PH_Beckhoff_PP_PU.evt Call PSU Inhibit off.vi"("i ref in"=w209, "PU"=w205, "error in"=w207) -> ("i ref out"=w208:refnum<vi>, "error out"=w206:errorcluster)  [unwired: 15 in]
          }
          frame True {
            n102 = call "PH_Beckhoff_PP_PU.evt Call PSU Inhibit on.vi"("i ref in"=w214, "PU"=w210, "error in"=w212) -> ("i ref out"=w213:refnum<vi>, "error out"=w211:errorcluster)  [unwired: 15 in]
          }
        }
        n103 = property on="_inhibit_on PSU 1" class="Bool (strict)"(error in=w203, "Value"=w201) -> (error out=w202:errorcluster)  [unwired: 1 in, 1 out]
      }
      event "_inhibit_on PSU 2": Value Change {
        n104 = event-data() -> ("NewVal"=w225:bool, "OldVal"=w227:bool)  [unwired: 1 in]
        n105 = call "PH_Beckhoff_PP_PU.get PU Rack Type.vi"("VI in"=w219, "error in (no error)"=w218) -> ("VI out"=w216:refnum<vi>, "PU Rack Type"=w222:T11, "error out"=w217:errorcluster)  [unwired: 15 in]
        n106 = call "PH_Beckhoff_PP_PU.convert PU Type to PUs.vi"("PU Type"=w222) -> ("PUs"=w221:T22[])
        n107 = Index Array(array=w221, index=1) -> (element=w215:T22)
        n108 = case shown="True" w225 {
          tunnel: w216 -> [w232 w237]
          tunnel: [w231 w236] -> w224
          tunnel: w217 -> [w230 w235]
          tunnel: [w229 w234] -> w223
          tunnel: w215 -> [w228 w233]
          frame False {
            n109 = call "PH_Beckhoff_PP_PU.evt Call PSU Inhibit off.vi"("i ref in"=w232, "PU"=w228, "error in"=w230) -> ("i ref out"=w231:refnum<vi>, "error out"=w229:errorcluster)  [unwired: 15 in]
          }
          frame True {
            n110 = call "PH_Beckhoff_PP_PU.evt Call PSU Inhibit on.vi"("i ref in"=w237, "PU"=w233, "error in"=w235) -> ("i ref out"=w236:refnum<vi>, "error out"=w234:errorcluster)  [unwired: 15 in]
          }
        }
        n111 = property on="_inhibit_on PSU 2" class="Bool (strict)"(error in=w223, "Value"=w227) -> (error out=w226:errorcluster)  [unwired: 1 in, 1 out]
      }
      event "_interlock_on PSU 1": Value Change {
        n112 = event-data() -> ("NewVal"=w245:bool, "OldVal"=w249:bool)  [unwired: 1 in]
        n113 = call "PH_Beckhoff_PP_PU.get PU Rack Type.vi"("VI in"=w242, "error in (no error)"=w241) -> ("VI out"=w240:refnum<vi>, "PU Rack Type"=w244:T11, "error out"=w239:errorcluster)  [unwired: 15 in]
        n114 = call "PH_Beckhoff_PP_PU.convert PU Type to PUs.vi"("PU Type"=w244) -> ("PUs"=w243:T22[])
        n115 = Index Array(array=w243) -> (element=w238:T22)  [unwired: 1 in]
        n116 = case shown="True" w245 {
          tunnel: w239 -> [w252 w259]
          tunnel: w240 -> [w254 w258]
          tunnel: [w251 w257] -> w247
          tunnel: [w253 w256] -> w246
          tunnel: w238 -> [w250 w255]
          frame False {
            n117 = call "PH_Beckhoff_PP_PU.evt Call PSU Interlock off.vi"("i ref in"=w254, "PU"=w250, "error in"=w252) -> ("i ref out"=w253:refnum<vi>, "error out"=w251:errorcluster)  [unwired: 15 in]
          }
          frame True {
            n118 = call "PH_Beckhoff_PP_PU.evt Call PSU Interlock on.vi"("i ref in"=w258, "PU"=w255, "error in"=w259) -> ("i ref out"=w256:refnum<vi>, "error out"=w257:errorcluster)  [unwired: 15 in]
          }
        }
        n119 = property on="_interlock_on PSU 1" class="Bool (strict)"(error in=w247, "Value"=w249) -> (error out=w248:errorcluster)  [unwired: 1 in, 1 out]
      }
      event "_interlock_on PSU 2": Value Change {
        n120 = event-data() -> ("NewVal"=w270:bool, "OldVal"=w272:bool)  [unwired: 1 in]
        n121 = call "PH_Beckhoff_PP_PU.get PU Rack Type.vi"("VI in"=w264, "error in (no error)"=w263) -> ("VI out"=w262:refnum<vi>, "PU Rack Type"=w267:T11, "error out"=w261:errorcluster)  [unwired: 15 in]
        n122 = call "PH_Beckhoff_PP_PU.convert PU Type to PUs.vi"("PU Type"=w267) -> ("PUs"=w266:T22[])
        n123 = Index Array(array=w266, index=1) -> (element=w260:T22)
        n124 = case shown="True" w270 {
          tunnel: w261 -> [w275 w282]
          tunnel: w262 -> [w277 w281]
          tunnel: [w274 w280] -> w269
          tunnel: [w276 w279] -> w268
          tunnel: w260 -> [w273 w278]
          frame False {
            n125 = call "PH_Beckhoff_PP_PU.evt Call PSU Interlock off.vi"("i ref in"=w277, "PU"=w273, "error in"=w275) -> ("i ref out"=w276:refnum<vi>, "error out"=w274:errorcluster)  [unwired: 15 in]
          }
          frame True {
            n126 = call "PH_Beckhoff_PP_PU.evt Call PSU Interlock on.vi"("i ref in"=w281, "PU"=w278, "error in"=w282) -> ("i ref out"=w279:refnum<vi>, "error out"=w280:errorcluster)  [unwired: 15 in]
          }
        }
        n127 = property on="_interlock_on PSU 2" class="Bool (strict)"(error in=w269, "Value"=w272) -> (error out=w271:errorcluster)  [unwired: 1 in, 1 out]
      }
      event "_HV_on PSU 1": Value Change {
        n128 = event-data() -> ("NewVal"=w290:bool, "OldVal"=w293:bool)  [unwired: 1 in]
        n129 = call "PH_Beckhoff_PP_PU.get PU Rack Type.vi"("VI in"=w287, "error in (no error)"=w286) -> ("VI out"=w285:refnum<vi>, "PU Rack Type"=w289:T11, "error out"=w284:errorcluster)  [unwired: 15 in]
        n130 = call "PH_Beckhoff_PP_PU.convert PU Type to PUs.vi"("PU Type"=w289) -> ("PUs"=w288:T22[])
        n131 = Index Array(array=w288) -> (element=w283:T22)  [unwired: 1 in]
        n132 = case shown="True" w290 {
          tunnel: w285 -> [w299 w304]
          tunnel: w284 -> [w297 w303]
          tunnel: [w298 w302] -> w292
          tunnel: [w296 w301] -> w291
          tunnel: w283 -> [w295 w300]
          frame False {
            n133 = call "PH_Beckhoff_PP_PU.evt Call PSU HV off.vi"("i ref in"=w299, "PU"=w295, "error in"=w297) -> ("i ref out"=w298:refnum<vi>, "error out"=w296:errorcluster)  [unwired: 15 in]
          }
          frame True {
            n134 = call "PH_Beckhoff_PP_PU.evt Call PSU HV on.vi"("i ref in"=w304, "PU"=w300, "error in"=w303) -> ("i ref out"=w302:refnum<vi>, "error out"=w301:errorcluster)  [unwired: 15 in]
          }
        }
        n135 = property on="_HV_on PSU 1" class="Bool (strict)"(error in=w291, "Value"=w293) -> (error out=w294:errorcluster)  [unwired: 1 in, 1 out]
      }
      event "_HV_on PSU 2": Value Change {
        n136 = event-data() -> ("NewVal"=w315:bool, "OldVal"=w317:bool)  [unwired: 1 in]
        n137 = call "PH_Beckhoff_PP_PU.get PU Rack Type.vi"("VI in"=w309, "error in (no error)"=w308) -> ("VI out"=w307:refnum<vi>, "PU Rack Type"=w312:T11, "error out"=w306:errorcluster)  [unwired: 15 in]
        n138 = call "PH_Beckhoff_PP_PU.convert PU Type to PUs.vi"("PU Type"=w312) -> ("PUs"=w311:T22[])
        n139 = Index Array(array=w311, index=1) -> (element=w305:T22)
        n140 = case shown="True" w315 {
          tunnel: w307 -> [w322 w327]
          tunnel: w306 -> [w320 w326]
          tunnel: [w321 w325] -> w313
          tunnel: [w319 w324] -> w314
          tunnel: w305 -> [w318 w323]
          frame False {
            n141 = call "PH_Beckhoff_PP_PU.evt Call PSU HV off.vi"("i ref in"=w322, "PU"=w318, "error in"=w320) -> ("i ref out"=w321:refnum<vi>, "error out"=w319:errorcluster)  [unwired: 15 in]
          }
          frame True {
            n142 = call "PH_Beckhoff_PP_PU.evt Call PSU HV on.vi"("i ref in"=w327, "PU"=w323, "error in"=w326) -> ("i ref out"=w325:refnum<vi>, "error out"=w324:errorcluster)  [unwired: 15 in]
          }
        }
        n143 = property on="_HV_on PSU 2" class="Bool (strict)"(error in=w314, "Value"=w317) -> (error out=w316:errorcluster)  [unwired: 1 in, 1 out]
      }
      event "_reset PSU 1": Value Change {
        n144 = event-data() -> ("NewVal"=w339:bool, "OldVal"=w335:bool)  [unwired: 1 in]
        n145 = call "PH_Beckhoff_PP_PU.get PU Rack Type.vi"("VI in"=w332, "error in (no error)"=w331) -> ("VI out"=w330:refnum<vi>, "PU Rack Type"=w334:T11, "error out"=w329:errorcluster)  [unwired: 15 in]
        n146 = call "PH_Beckhoff_PP_PU.convert PU Type to PUs.vi"("PU Type"=w334) -> ("PUs"=w333:T22[])
        n147 = Index Array(array=w333) -> (element=w328:T22)  [unwired: 1 in]
        n148 = case shown="False" w339 {
          tunnel: w330 -> [w344 w349]
          tunnel: w329 -> [w342 w348]
          tunnel: [w343 w347] -> w338
          tunnel: [w341 w346] -> w337
          tunnel: w328 -> [w340 w345]
          frame False {
            n149 = call "PH_Beckhoff_PP_PU.evt Call reset off.vi"("i ref in"=w344, "PU"=w340, "error in"=w342) -> ("i ref out"=w343:refnum<vi>, "error out"=w341:errorcluster)  [unwired: 15 in]
          }
          frame True {
            n150 = call "PH_Beckhoff_PP_PU.evt Call reset on.vi"("i ref in"=w349, "PU"=w345, "error in"=w348) -> ("i ref out"=w347:refnum<vi>, "error out"=w346:errorcluster)  [unwired: 15 in]
          }
        }
        n151 = property on="_reset PSU 1" class="Bool (strict)"(error in=w337, "Value"=w335) -> (error out=w336:errorcluster)  [unwired: 1 in, 1 out]
      }
      event "_reset PSU 2": Value Change {
        n152 = event-data() -> ("NewVal"=w362:bool, "OldVal"=w358:bool)  [unwired: 1 in]
        n153 = call "PH_Beckhoff_PP_PU.get PU Rack Type.vi"("VI in"=w354, "error in (no error)"=w353) -> ("VI out"=w350:refnum<vi>, "PU Rack Type"=w357:T11, "error out"=w352:errorcluster)  [unwired: 15 in]
        n154 = call "PH_Beckhoff_PP_PU.convert PU Type to PUs.vi"("PU Type"=w357) -> ("PUs"=w356:T22[])
        n155 = Index Array(array=w356, index=1) -> (element=w351:T22)
        n156 = case shown="True" w362 {
          tunnel: w350 -> [w367 w372]
          tunnel: w352 -> [w365 w371]
          tunnel: [w366 w370] -> w361
          tunnel: [w364 w369] -> w360
          tunnel: w351 -> [w363 w368]
          frame False {
            n157 = call "PH_Beckhoff_PP_PU.evt Call reset off.vi"("i ref in"=w367, "PU"=w363, "error in"=w365) -> ("i ref out"=w366:refnum<vi>, "error out"=w364:errorcluster)  [unwired: 15 in]
          }
          frame True {
            n158 = call "PH_Beckhoff_PP_PU.evt Call reset on.vi"("i ref in"=w372, "PU"=w368, "error in"=w371) -> ("i ref out"=w370:refnum<vi>, "error out"=w369:errorcluster)  [unwired: 15 in]
          }
        }
        n159 = property on="_reset PSU 2" class="Bool (strict)"(error in=w360, "Value"=w358) -> (error out=w359:errorcluster)  [unwired: 1 in, 1 out]
      }
      event "_set_voltage PSU 1": Value Change {
        n160 = event-data() -> ("NewVal"=w384:dbl, "OldVal"=w387:dbl)  [unwired: 1 in]
        n161 = call "PH_Beckhoff_PP_PU.get i attribute.vi"("i ref in"=w376, "error in (no error)"=w378) -> ("i ref out"=w375:refnum<vi>, "i attribute"=w374:T23, "error out"=w377:errorcluster)  [unwired: 15 in]
        n162 = Unbundle By Name(w374) -> ("PSU Info.Limits 1 [V]"=w373:cluster{"Lower":dbl, "Upper":dbl})
        n163 = call "PH_Beckhoff_PP_PU.get PU Rack Type.vi"("VI in"=w375, "error in (no error)"=w377) -> ("VI out"=w380:refnum<vi>, "PU Rack Type"=w383:T11, "error out"=w381:errorcluster)  [unwired: 15 in]
        n164 = call "PH_Beckhoff_PP_PU.convert PU Type to PUs.vi"("PU Type"=w383) -> ("PUs"=w382:T22[])
        n165 = Index Array(array=w382) -> (element=w379:T22)  [unwired: 1 in]
        n166 = call "PH_Beckhoff_PP_PU.evt Call PSU set Voltage.vi"("i ref in"=w380, "PU"=w379, "Voltage to set [V]"=w384, "error in"=w381, "Limits [V]"=w373) -> ("i ref out"=w388:refnum<vi>, "error out"=w386:errorcluster)  [unwired: 13 in]
        n167 = property on="_set_voltage PSU 1" class="DigNum (strict)"(error in=w386, "Value"=w387) -> (error out=w385:errorcluster)  [unwired: 1 in, 1 out]
      }
      event "_set_voltage PSU 2": Value Change {
        n168 = event-data() -> ("NewVal"=w403:dbl, "OldVal"=w404:dbl)  [unwired: 1 in]
        n169 = call "PH_Beckhoff_PP_PU.get i attribute.vi"("i ref in"=w394, "error in (no error)"=w395) -> ("i ref out"=w397:refnum<vi>, "i attribute"=w396:T23, "error out"=w398:errorcluster)  [unwired: 15 in]
        n170 = Unbundle By Name(w396) -> ("PSU Info.Limits 2 [V]"=w391:cluster{"Lower":dbl, "Upper":dbl})
        n171 = call "PH_Beckhoff_PP_PU.get PU Rack Type.vi"("VI in"=w397, "error in (no error)"=w398) -> ("VI out"=w393:refnum<vi>, "PU Rack Type"=w400:T11, "error out"=w392:errorcluster)  [unwired: 15 in]
        n172 = call "PH_Beckhoff_PP_PU.convert PU Type to PUs.vi"("PU Type"=w400) -> ("PUs"=w399:T22[])
        n173 = Index Array(array=w399, index=1) -> (element=w390:T22)
        n174 = call "PH_Beckhoff_PP_PU.evt Call PSU set Voltage.vi"("i ref in"=w393, "PU"=w390, "Voltage to set [V]"=w403, "error in"=w392, "Limits [V]"=w391) -> ("i ref out"=w402:refnum<vi>, "error out"=w401:errorcluster)  [unwired: 13 in]
        n175 = property on="_set_voltage PSU 2" class="DigNum (strict)"(error in=w401, "Value"=w404) -> (error out=w405:errorcluster)  [unwired: 1 in, 1 out]
      }
      event User Event {
        n176 = event-data() -> ("Class"=w425:string)  [unwired: 1 in]
        n177 = case shown="\"PH_Beckhoff_PP_PU\"" w425 {
          selector: w425 -> [w430 _]
          tunnel: w428 -> [w434 w461]
          tunnel: w427 -> [w432 w460]
          tunnel: [w433 w444] -> w409
          tunnel: [w431 w443] -> w426
          tunnel: w424 -> [_ w459]
          tunnel: w423 -> [_ w458]
          tunnel: w422 -> [_ w457]
          tunnel: w421 -> [_ w456]
          tunnel: w420 -> [_ w455]
          tunnel: w419 -> [_ w454]
          tunnel: w418 -> [_ w453]
          tunnel: w417 -> [_ w452]
          tunnel: w416 -> [_ w451]
          tunnel: w415 -> [_ w450]
          tunnel: w414 -> [_ w449]
          tunnel: w413 -> [_ w448]
          tunnel: w412 -> [_ w447]
          tunnel: w411 -> [w429 _]
          tunnel: w407 -> [_ w439]
          tunnel: w406 -> [_ w438]
          frame Default {
            n178 = call "PH_Beckhoff.set GUI Refs.vi"("i ref in"=w434, "Class"=w430, "GUI Refs"=w429, "error in"=w432) -> ("i ref out"=w433:refnum<vi>, "error out"=w431:errorcluster)  [unwired: 14 in]
          }
          frame "PH_Beckhoff_PP_PU" {
            n179 = call "PH_Beckhoff_PP_PU.get data to modify.vi"("i ref in"=w461, "ms timeout (10000)"=-1, "error in (no error)"=w460) -> ("i ref out"=w474:refnum<vi>, "i attribute"=w473:T23, "error out"=w477:errorcluster)  [unwired: 13 in, 1 out]
            n180 = Unbundle By Name(w473) -> ("Igni"=w467:T27, "RR"=w468:T28, "Trigger"=w465:T29, "HV Meas"=w471:T30, "PSU"=w462:T31)
            n181 = for {
              tunnel: w453 -> [w524] mode=indexing
              tunnel: w462 -> [w526] mode=indexing
              tunnel: [w525] -> w463 mode=indexing
              tunnel: w452 -> [w510] mode=indexing
              tunnel: w451 -> [w509] mode=indexing
              tunnel: w450 -> [w508] mode=indexing
              tunnel: w449 -> [w507] mode=indexing
              tunnel: w448 -> [w506] mode=indexing
              n182 = property class="Clust (strict)"(reference=w524) -> (reference out=w505:refnum<vi>, "Controls[]"=w523:refnum<vi>[])  [unwired: 1 in, 1 out]
              n183 = Index Array(array=w523) -> (element #1=w522:refnum<vi>, element #2=w521:refnum<vi>, element #3=w520:refnum<vi>, element #4=w519:refnum<vi>, element #5=w518:refnum<vi>, element #6=w517:refnum<vi>, element #7=w516:refnum<vi>, element #8=w515:refnum<vi>, element #9=w514:refnum<vi>, element #10=w513:refnum<vi>, element #11=w512:refnum<vi>, element #12=w511:refnum<vi>)  [unwired: 12 in]
              n184 = Bundle By Name(cluster=w526, "GUI Ref Indicator"=w505, "Status.GUI Ref"=w522, "DIs.inhibit.GUI Ref"=w521, "DIs.end of charge.GUI Ref"=w520, "DIs.HV on.GUI Ref"=w519, "DIs.overtemp.GUI Ref"=w518, "DIs.interlock.GUI Ref"=w517, "DIs.load fault.GUI Ref"=w516, "DIs.sum fault.GUI Ref"=w515, "DIs.HV off.GUI Ref"=w514, "DIs.DC ok.GUI Ref"=w513, "AIs.voltage.GUI Ref"=w512, "AIs.current.GUI Ref"=w511, "DAs.inhibit.GUI Ref"=w510, "DAs.interlock.GUI Ref"=w509, "DAs.HV on.GUI Ref"=w508, "DAs.Reset.GUI Ref"=w507, "AAs.Voltage to set.GUI Ref"=w506) -> (w525:T32)
            }
            n185 = for {
              tunnel: [w504] -> w466 mode=indexing
              tunnel: w467 -> [w503] mode=indexing
              tunnel: w459 -> [w500] mode=indexing
              tunnel: w458 -> [w502] mode=indexing
              n186 = property class="Clust (strict)"(reference=w500) -> (reference out=w496:refnum<vi>, "Controls[]"=w501:refnum<vi>[])  [unwired: 1 in, 1 out]
              n187 = Index Array(array=w501) -> (element #1=w499:refnum<vi>, element #2=w498:refnum<vi>, element #3=w497:refnum<vi>)  [unwired: 3 in]
              n188 = Bundle By Name(cluster=w503, "GUI Ref Indicator"=w496, "Status.GUI Ref"=w499, "DIs.heating on.GUI Ref"=w498, "DIs.water on.GUI Ref"=w497, "Device on.GUI Ref"=w502) -> (w504:T33)
            }
            n189 = for {
              tunnel: [w495] -> w469 mode=indexing
              tunnel: w468 -> [w494] mode=indexing
              tunnel: w456 -> [w493] mode=indexing
              tunnel: w457 -> [w492] mode=indexing
              n190 = property class="Clust (strict)"(reference=w492) -> (reference out=w487:refnum<vi>, "Controls[]"=w491:refnum<vi>[])  [unwired: 1 in, 1 out]
              n191 = Index Array(array=w491) -> (element #1=w488:refnum<vi>, element #2=w489:refnum<vi>, element #3=w490:refnum<vi>)  [unwired: 3 in]
              n192 = Bundle By Name(cluster=w494, "GUI Ref Indicator"=w487, "Status.GUI Ref"=w488, "DIs.closed.GUI Ref"=w489, "DIs.open.GUI Ref"=w490, "Close.GUI Ref"=w493) -> (w495:T34)
            }
            n193 = for {
              tunnel: w455 -> [w486] mode=indexing
              tunnel: w465 -> [w485] mode=indexing
              tunnel: [w484] -> w464 mode=indexing
              n194 = property class="Clust (strict)"(reference=w486) -> (reference out=w478:refnum<vi>, "Controls[]"=w483:refnum<vi>[])  [unwired: 1 in, 1 out]
              n195 = Index Array(array=w483) -> (element #1=w482:refnum<vi>, element #2=w481:refnum<vi>, element #3=w480:refnum<vi>, element #4=w479:refnum<vi>)  [unwired: 4 in]
              n196 = Bundle By Name(cluster=w485, "GUI Ref Indicator"=w478, "Status.GUI Ref"=w482, "DIs.triggered.GUI Ref"=w481, "DIs.fired.GUI Ref"=w480, "last shot:.GUI Ref"=w479) -> (w484:T35)
            }
            n197 = for {
              tunnel: w454 -> [w529] mode=indexing
              tunnel: w471 -> [w528] mode=indexing
              tunnel: [w527] -> w470 mode=indexing
              n198 = Bundle By Name(cluster=w528, "Input GUI Ref"=w529) -> (w527:T36)
            }
            n199 = Bundle By Name(cluster=w473, "Igni"=w466, "RR"=w469, "Trigger"=w464, "HV Meas"=w470, "PSU"=w463, "reconfigured.GUI Ref"=w447) -> (w437:T23)
            n200 = call "PH_Beckhoff_PP_PU.set modified data.vi"("i ref in"=w474, "i attribute"=w437, "error in (no error)"=w477) -> ("i ref out"=w472:refnum<vi>, "error out"=w475:errorcluster)  [unwired: 15 in]
            n201 = call "PH_Beckhoff_PP_PU.set GUI Elements to Default.vi"("i ref in"=w472, "error in"=w475) -> ("i ref out"=w436:refnum<vi>, "error out"=w435:errorcluster)  [unwired: 16 in]
            n202 = Unbundle By Name(w437) -> ("PSU Info.Limits 1 [V]"=→"Limits 1 [V]":cluster{"Lower":dbl, "Upper":dbl}, "PSU Info.Limits 2 [V]"=→"Limits 2 [V]":cluster{"Lower":dbl, "Upper":dbl})
            n203 = call "PH_Beckhoff_PP_PU.set further GUI Objects.vi"("VI in"=w436, "Refs HV Meas"=w438, "Refs Voltage"=w439, "error in (no error)"=w435) -> ("VI out"=w444:refnum<vi>, "Type PSU 1"=→"Type PSU 1":T17, "Type PSU 2"=→"Type PSU 2":T17, "PU Rack Type"=→"PU Rack Type":T11, "error out"=w443:errorcluster)  [unwired: 11 in]
          }
        }
        n204 = call "PH_Class.set GUI Refs stored Occurence.vi"("i ref in"=w409, "error in (no error)"=w426) -> ("i ref out"=w408:refnum<vi>, "error out"=w410:errorcluster)  [unwired: 16 in]
      }
    }
  }
  "error out" <- w58
  n205 = call "PH_Interaction.Super Destroy Me.vi"("i ref out"=w59) -> ()
  n206 = Unregister For Events(event registration refnum=w21) -> ()  [unwired: 1 in, 1 out]
